vi "add_uint16_roslv.vi"   [LabVIEW 2014]
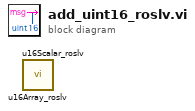
[diagram p0: block diagram]
diagram:
  n1 = call "u16Array_roslv.vi"() -> ()  [unwired: 5 in, 1 out]
  n2 = call "u16Scalar_roslv.vi"() -> ()  [unwired: 5 in, 1 out]
